vi "UDP Listener.vi"() -> ()   [LabVIEW 2009]
uses:
  <vilib>/Platform/TimedLoop/XDataNode/XDataNode.xnode
  <vilib>/Platform/TimedLoop/XDataNode/loadlvalarms.vi
  <vilib>/Platform/TimedLoop/XDataNode/timing_clust.ctl
  <vilib>/Platform/TimedLoop/XDataNode/nitl_modes.ctl
  <vilib>/Platform/TimedLoop/XDataNode/wakeup.ctl
  <vilib>/Platform/TimedLoop/XDataNode/XDNodeRunTimeDep.lvlib
panel:
  out "Receive Data":string
  in  "stop":bool
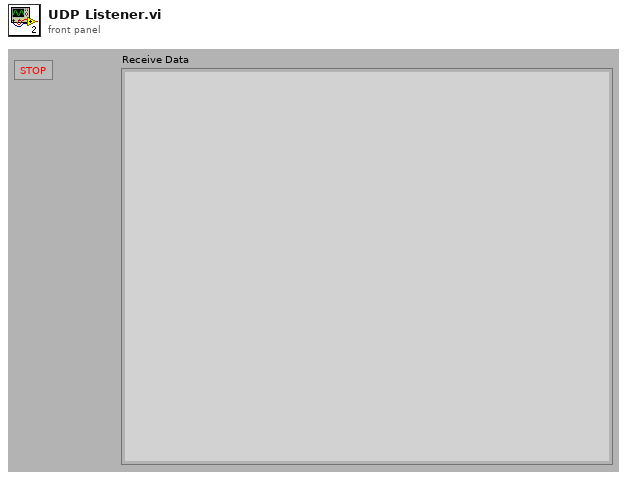
[diagram p1: front panel]
types:
  T1 = typedef "UDP Base.ctl" = cluster{"UDP Session":refnum<k16>, "UDP Socket Params":T2}
  T2 = typedef "UDP Socket Params.ctl" = cluster{"Local Port":u16, "Read Timeout":i32, "Write Timeout":i32}
  T3 = typedef "XDNodeRunTimeDep.lvlib/timing_clust.ctl" = cluster{"Expected End [f-1]":u64, "Actual End [f-1]":u64, "Finished Late? [f-1]":bool, "Expected End [i-1]":u64, "Actual End [i-1]":u64, "Finished Late? [i-1]":bool, "Expected Start [i]":u64, "Actual Start [i]":u64, "Expected Start [f]":u64, "Actual Start [f]":u64, "Source Name":string, "Structure Name":string, "Period":i64, "Deadline":i64, "Offset":i64, "Start":i64, "Priority":i32, "Timeout":i32, "Mode":T4, "Wakeup Reason":T5, "Error":errorcluster, "Source Type":string, "Secondary Source Type":string, "Global End Time":u64, "Global Start Time":u64, "Frame Duration":u64, "Iteration Duration":u64, "Assigned CPU":i32, "I/O Scan Engine Mode":u32}
  T4 = typedef "XDNodeRunTimeDep.lvlib/nitl_modes.ctl" = enum32{"No Change", "Process missed periods, maintain original phase", "Discard missed periods, maintain original phase", "Process missed periods, ignore original phase", "Discard missed periods, ignore original phase"}
  T5 = typedef "XDNodeRunTimeDep.lvlib/wakeup.ctl" = enum32{"Normal", "Aborted", "Asynchronous wakeup", "Timing source error", "Timed loop error", "Timeout"}
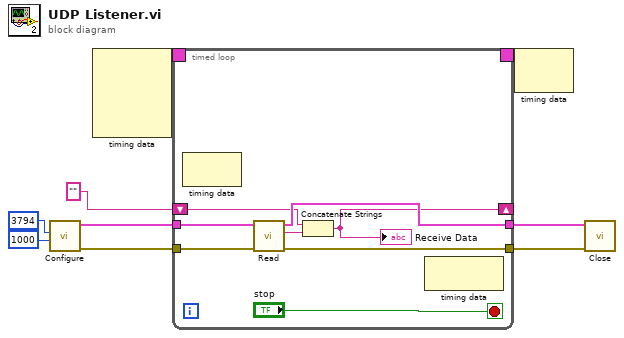
[diagram p0: block diagram]
diagram:
  n1 = call "Configure.vi"("Read Timeout"=1000, "Local Port"=u16 3794) -> ("error out"=w7:errorcluster, "UDP Base out"=w6:T1)  [unwired: 8 in]
  n2 = node-c288() -> (w9:T3)  [unwired: 4 in]
  n3 = timed-loop {
    timing: w9 -> [_]
    timing-out: [_] -> w8
    tunnel: w7 -> [w16]
    tunnel: w6 -> [w15]
    tunnel: [w14] -> w5
    tunnel: [w13] -> w4
    shift-right: [w10] -> _
    shift-left: "" -> [w11]
    stop <- "stop" stop-if-true
    n4 = node-c288() -> ()  [unwired: 1 in, 1 out]
    n5 = call "Read.vi"("error in (no error)"=w16, "UDP Base in"=w15) -> ("error out"=w13:errorcluster, "Receive Data"=w12:string, "UDP Base out"=w14:T1)  [unwired: 4 in, 3 out]
    n6 = Concatenate Strings(w11, w12) -> (w10:string)
    "Receive Data" <- w10
    n7 = node-c288() -> ()  [unwired: 1 in, 1 out]
  }
  n8 = node-c288(w8) -> ()  [unwired: 1 out]
  n9 = call "Close.vi"("error in (no error)"=w4, "Cluster of class private data"=w5) -> ()  [unwired: 9 in, 1 out]
